vi "AA_CLock_3.vi"() -> ()   [LabVIEW 2019]
doc: "A vi that represents a clock with seconds-minutes-hours hands.\n\nBored? is used to make time faster starting from current time and increasing time by the rate of loop index."
panel:
  out "Second":sgl(knob) scale=0.0..60.0
  out "Minute":sgl(knob) scale=0.0..60.0
  out "Hour":sgl(knob) scale=0.0..12.0
  out "Dial":sgl(knob) scale=0.0..12.0
  out "Time Indicator":timestamp format="%<%X>T"
  out "Clock":T1 {"Seconds 2" scale=0.0..60.0; "Hours 2" scale=0.0..24.0; "Minutes 2" scale=0.0..60.0}
  in  "Bored?":bool
  in  "STOP":bool
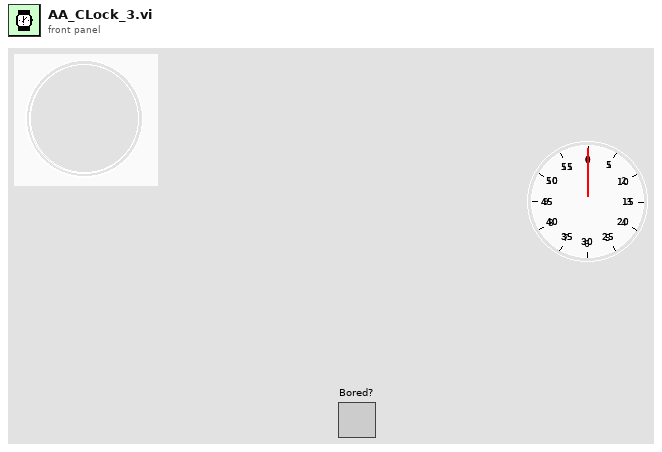
[diagram p1: front panel]
types:
  T1 = cluster{"Minutes 2":sgl, "Hours 2":sgl, "Seconds 2":sgl}
  T2 = typedef "LVDateTimeRec.ctl" = cluster{"fractional second":dbl, "second":i32, "minute":i32, "hour":i32, "day of month":i32, "month":i32, "year":i32, "day of week":i32, "day of year":i32, "DST":i32}
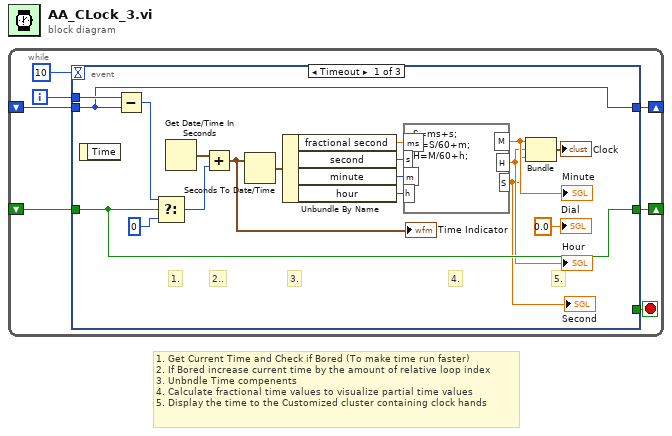
[diagram p0: block diagram]
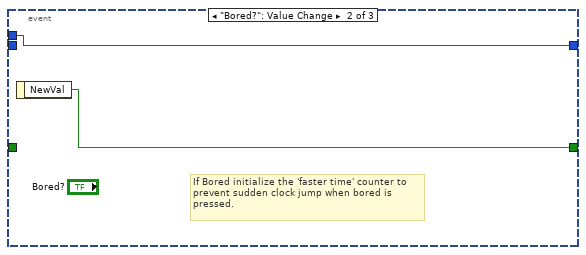
[diagram p2: hidden frame]
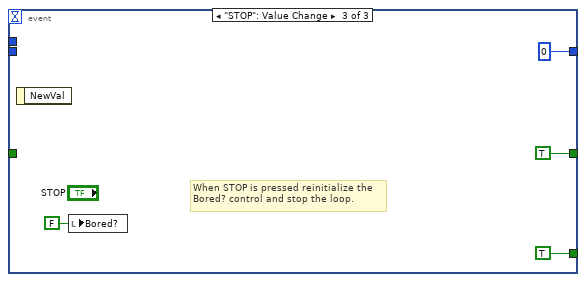
[diagram p3: hidden frame]
diagram:
  # "1. Get Current Time and Check if Bored (To make time run faster)\n2. If Bored increase current time by the amount of relative loop index\n3. Unbndle Time compenents\n4. Calculate fractional time values to visualize partial time values\n5. Display the time to the Customized cluster containing clock hands"
  n1 = while {
    shift-right: [w5] -> _
    shift-left: _ -> [w4]
    shift-right: [w3] -> _
    shift-left: _ -> [w1]
    i -> [w2]
    stop <- w6 stop-if-true
    n2 = event shown="[0] Timeout" {
      selector: _ -> [_ _ _]
      dyn-events: _ -> [_ _ _]
      timeout: 10 -> [_ _ _]
      tunnel: [_ _ TRUE] -> w6
      tunnel: [w25 w27 TRUE ("NewVal")] -> w5
      tunnel: w4 -> [w25 _ _]
      tunnel: [w23 w26 0] -> w3
      tunnel: w2 -> [w24 w26 _]
      tunnel: w1 -> [w23 _ _]
      event Timeout {
        # "5."
        # "4."
        # "3."
        # "2.."
        # "1."
        n3 = event-data() -> ()  [unwired: 1 in, 1 out]
        n4 = Subtract(x=w24, y=w23) -> (x-y=w22:i32)
        n5 = Select(t=w22, s=w25, f=0) -> (s? t:f=w14:i32)
        n6 = Get Date/Time In Seconds() -> (seconds since 1Jan1904=w16:timestamp)
        n7 = Add(x=w16, y=w14) -> (x+y=w12:timestamp)
        "Time Indicator" <- w12
        n8 = Seconds To Date/Time(time stamp (now)=w12) -> (date time rec=w15:T2)  [unwired: 1 in]
        n9 = Unbundle By Name(w15) -> ("fractional second"=w17:dbl, "second"=w18:i32, "minute"=w19:i32, "hour"=w20:i32)
        n10 = formula code="S=ms+s;\nM=S/60+m;\nH=M/60+h;"("ms"=w17, "s"=w18, "m"=w19, "h"=w20) -> ("M"=w10:dbl, "H"=w9:dbl, "S"=w8:dbl)
        "Hour" <- w9
        "Minute" <- w10
        "Second" <- w8
        n11 = Bundle("M"=w10, "H"=w9, "S"=w8) -> (→"Clock":cluster{"M":dbl, "H":dbl, "S":dbl})  [unwired: 1 in]
        "Dial" <- sgl 0.0 ("Dial")
      }
      event "Bored?": Value Change {
        # "If Bored initialize the 'faster time' counter to\nprevent sudden clock jump when bored is \npressed."
        n12 = event-data() -> ("NewVal"=w27:bool)  [unwired: 1 in]
      }
      event "STOP": Value Change {
        # "When STOP is pressed reinitialize the\nBored? control and stop the loop."
        n13 = event-data() -> ()  [unwired: 1 in, 1 out]
        n14 = local write "Bored?"(FALSE ("Bored?")) -> ()
      }
    }
  }
